vi "Write Command and Read Response.vi"(8 "error in (no error)":errorcluster, 9 "milliseconds to wait":u32=100, 10 "Serial Command":string, 11 "VISA Refnum in":refnum<visa-resource-name>) -> (0 "error out":errorcluster, 2 "Line Feed Separated Response":string[](array[string]), 3 "VISA Refnum out":refnum<visa-resource-name>)   [LabVIEW 2018]
doc: "Writes a <b>Serial Command</b> to the NI-VISA Serial Buffer and accumulates all response data characters from the connected serial device, and passes them through the <b>Line Feed Separated Response</b> array."
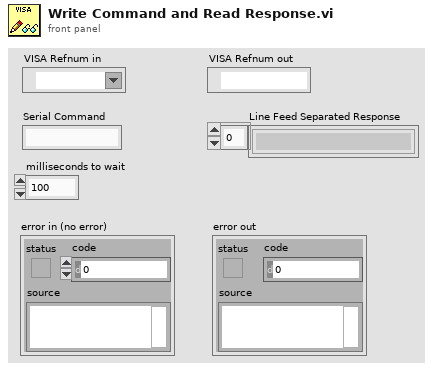
[diagram p1: front panel]
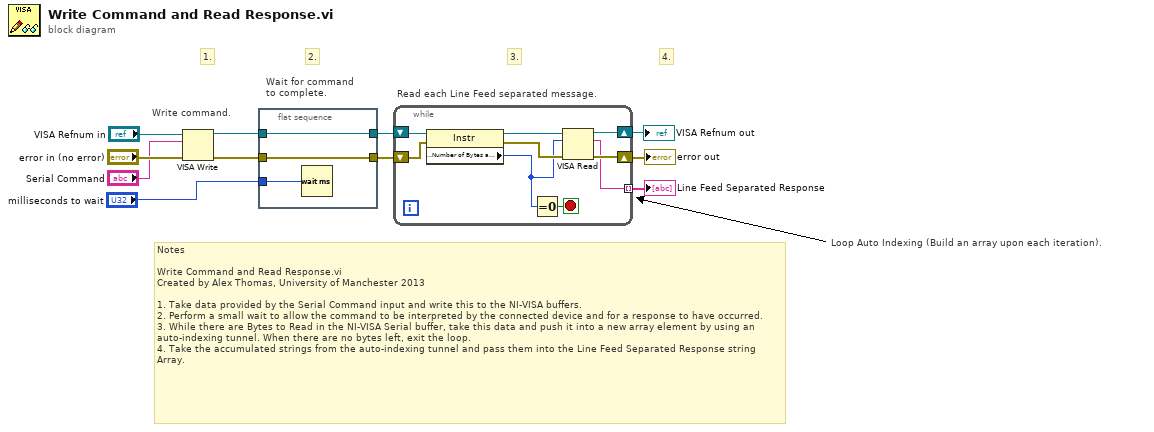
[diagram p0: block diagram]
diagram:
  # "Loop Auto Indexing (Build an array upon each iteration)."
  # "Notes\n\nWrite Command and Read Response.vi\nCreated by Alex Thomas, University of Manchester 2013\n\n1. Take data provided by the Serial Command input and write this to the NI-VISA buffers.\n2. Perform a small wait to allow the command to be interpreted by the connected device and for a response to have occurred. \n3. While there are Bytes to Read in the NI-VISA Serial buffer, take this data and push it into a new array element by using an auto-indexing tunnel. When there are no bytes left, exit the loop.\n4. Take the accumulated strings from the auto-indexing tunnel and pass them into the Line Feed Separated Response string Array."
  # "4."
  # "3."
  # "2."
  # "1."
  # "Read each Line Feed separated message."
  # "Wait for command\nto complete."
  # "Write command."
  n1 = VISA Write(VISA resource name="VISA Refnum in", write buffer="Serial Command", error in (no error)="error in (no error)") -> (VISA resource name out=w6:refnum<visa-resource-name>, error out=w8:errorcluster)  [unwired: 1 out]
  n2 = flat-sequence {
    tunnel: [w14] -> w5
    tunnel: w6 -> [w14]
    tunnel: [w13] -> w7
    tunnel: w8 -> [w13]
    tunnel: "milliseconds to wait" -> [w12]
    frame #0 {
      n3 = Wait (ms)(milliseconds to wait=w12) -> ()  [unwired: 1 out]
    }
  }
  n4 = while {
    shift-right: [w17] -> w10
    shift-left: w7 -> [w22]
    shift-right: [w16] -> w9
    shift-left: w5 -> [w23]
    tunnel: [w15] -> w11 mode=indexing
    stop <- w21 stop-if-true
    n5 = property class="Instr"(reference=w23, error in=w22) -> (reference out=w20:refnum<visa-resource-name>, error out=w19:errorcluster, "Serial Settings:Number of Bytes at Serial Port"=w18:u32)
    n6 = Equal To 0?(x=w18) -> (x = 0?=w21:bool)
    n7 = VISA Read(VISA resource name=w20, byte count=w18, error in (no error)=w19) -> (VISA resource name out=w16:refnum<visa-resource-name>, read buffer=w15:string, error out=w17:errorcluster)  [unwired: 1 out]
  }
  "Line Feed Separated Response" <- w11
  "error out" <- w10
  "VISA Refnum out" <- w9
